vi "pf_Init.vi"(8 "error in (no error)":errorcluster, 11 "Interface Name":string="img0::0") -> (0 "error out":errorcluster, 3 "IMAQ Session out":refnum<k11>)   [LabVIEW 2025, in "Photonfocus_Toolkit.lvlib"]
doc: "Initializes communication with the camera."
uses:
  Photonfocus_Toolkit.lvlib
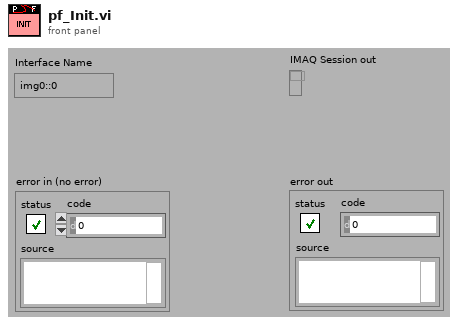
[diagram p1: front panel]
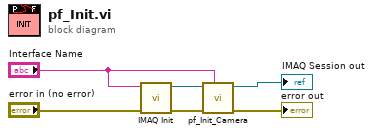
[diagram p0: block diagram]
diagram:
  n1 = call <vilib>:"IMAQ Init.vi"("error in (no error)"="error in (no error)", "Interface Name"="Interface Name") -> ("error out"=w6:errorcluster, "IMAQ Session Out"=w3:refnum<k11>)  [unwired: 8 out]
  n2 = call "pf_Init_Camera.vi"("Interface Name"="Interface Name", "error in (no error)"=w6, "IMAQ Session in"=w3) -> ("error out"=→"error out":errorcluster, "IMAQ Session out"=→"IMAQ Session out":refnum<k11>)  [unwired: 1 in, 6 out]
